vi "TCP Check Connection.vi"(8 "error in":errorcluster, 11 "connection in":T1) -> (0 "error out":errorcluster, 2 "disconnected?":bool, 3 "connection out":T1)   [LabVIEW 2010, in "NI STM.lvlib"]
doc: "This VI removes the host connection from the connection manager list if it becomes disconnected for any reason.\n\nCopyright 2015, 2016, 2017 National Instruments Corporation\n\nLicensed under the Apache License, Version 2.0 (the \"License\"); you may not use this file except in compliance with the License.\n\n You may obtain a copy of the License at\n\n http://www.apache.org/licenses/LICENSE-2.0\n\nUnless required by applicable law or agreed to in writing, software distributed under the License is distributed on an \"AS IS\" BASIS, WITHOUT WARRANTIES OR CONDITIONS OF ANY KIND, either express or implied.\n\nSee the License for the specific language governing permissions and limitations under the License."
uses:
  NI STM.lvlib
  TCP/TCP Connection Info.ctl
  SubVIs/MetaDataElement.ctl
  TCP Connection Method.ctl
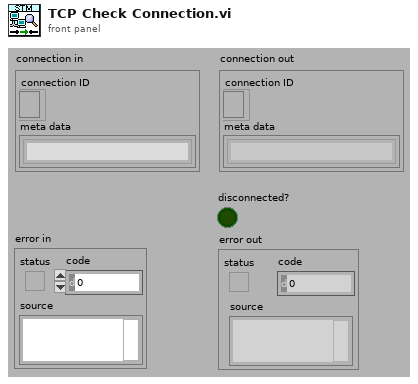
[diagram p1: front panel]
types:
  T1 = typedef "NI STM.lvlib/TCP Connection Info.ctl" = cluster{"connection ID":refnum<k5>, "meta data":T2[]}
  T2 = typedef "NI STM.lvlib/MetaDataElement.ctl" = string
  T3 = typedef "NI STM.lvlib/TCP Connection Method.ctl" = enum16{"Initialize", "Add Connection", "Set Properties", "Get Connection(s)", "Remove Connection", "Remove All Connections", "Get Connection Count"}
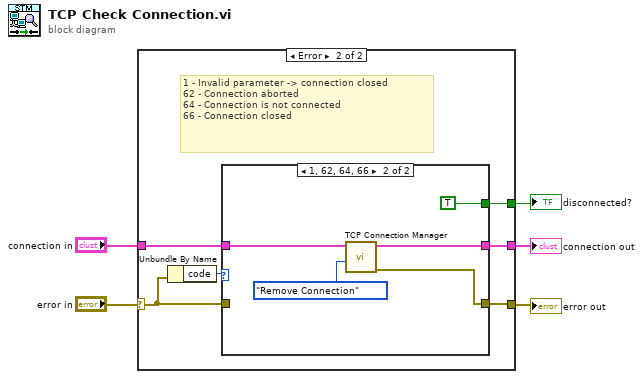
[diagram p0: block diagram]
diagram:
  n1 = case shown="Error" "error in" {
    selector: "error in" -> [w7 w12]
    tunnel: [w7 w11] -> w4
    tunnel: "connection in" -> [w6 w10]
    tunnel: [w6 w9] -> w2
    tunnel: [_ w8] -> w1
    frame No Error {
    }
    frame Error {
      # "1 - Invalid parameter -> connection closed\n62 - Connection aborted\n64 - Connection is not connected\n66 - Connection closed"
      n2 = Unbundle By Name(w12) -> ("code"=w13:i32)
      n3 = case shown="1, 62, 64, 66" w13 {
        tunnel: w12 -> [w15 _]
        tunnel: [w15 w18] -> w11
        tunnel: w10 -> [w14 w17]
        tunnel: [w14 w16] -> w9
        tunnel: [_ TRUE] -> w8
        frame Default {
        }
        frame 1, 62, 64, 66 {
          n4 = call "TCP Connection Manager.vi"("method"=TCP_Connection_Method."Remove Connection" ("Method"), "connection in"=w17) -> ("error out"=w18:errorcluster, "connection out"=w16:T1)  [unwired: 3 in, 5 out]
        }
      }
    }
  }
  "error out" <- w4
  "connection out" <- w2
  "disconnected?" <- w1
